vi "Outward Local Transition.vi"(8 "error in (no error)":errorcluster, 9 "Target State":refnum<class "State.lvclass">, 10 "Context in":refnum<class "Context.lvclass">, 11 "State in":refnum<class "State.lvclass">) -> (0 "error out":errorcluster, 2 "Context out":refnum<class "Context.lvclass">, 3 "State out":refnum<class "State.lvclass">)   [LabVIEW 2024, in "State.lvlib" / "State.lvclass"]
uses:
  State.lvclass
  Context/Context/Context.lvclass
  Container State/Container State.lvclass
  State.lvclass/State.ctl
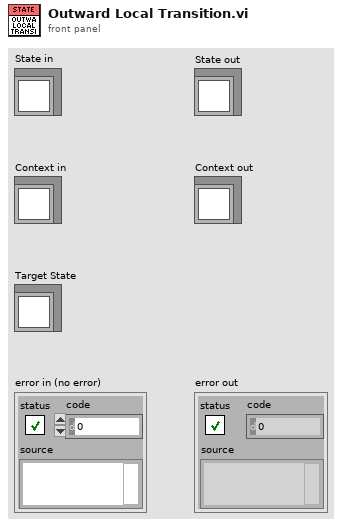
[diagram p1: front panel]
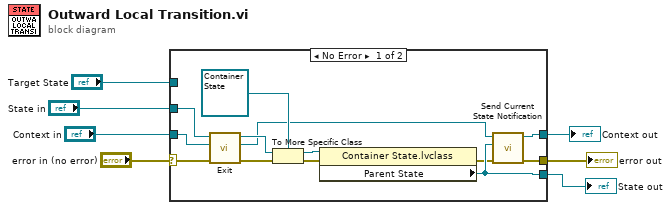
[diagram p0: block diagram]
diagram:
  n1 = case shown="No Error" "error in (no error)" {
    selector: "error in (no error)" -> [w19 w23]
    tunnel: [w8 w23] -> w6
    tunnel: [w11 w22] -> w2
    tunnel: "State in" -> [w13 w22]
    tunnel: [w10 w21] -> w4
    tunnel: "Context in" -> [w20 w21]
    tunnel: "Target State" -> [_ _]
    frame No Error {
      n2 = call-dynamic "Exit.vi"("error in (no error)"=w19, "Context in"=w20, "State in"=w13) -> ("error out"=w15:errorcluster, "Context out"=w12:refnum<class "Context.lvclass">, "State out"=w17:refnum<class "State.lvclass">)  [unwired: 6 in]
      n3 = To More Specific Class(target class=refnum<class "Container State.lvclass"> refnum ("State.lvlib:Container State.lvclass"), reference=w17, error in=w15) -> (specific class reference=w16:refnum<class "Container State.lvclass">, error out=w14:errorcluster)
      n4 = property class="Container State.lvclass"(reference=w16, error in=w14) -> (error out=w9:errorcluster, "Parent State"=w11:refnum<class "State.lvclass">)  [unwired: 1 out]
      n5 = call "Send Current State Notification.vi"("error in (no error)"=w9, "State"=w11, "Context in"=w12) -> ("error out"=w8:errorcluster, "Context out"=w10:refnum<class "Context.lvclass">)  [unwired: 7 in]
    }
    frame Error {
    }
  }
  "error out" <- w6
  "Context out" <- w4
  "State out" <- w2
